vi "IHM_detection_powerSpectrum.vi"() -> ()   [LabVIEW 2009]
uses:
  <vilib>/Analysis/4window.llb/windowTd.ctl
  <vilib>/measure/maspectr.llb/FFT Power Spectrum for 1 Chan.vi
  <vilib>/measure/NI_MAPro.lvlib
  <vilib>/Analysis/NI_AALPro.lvlib
  <vilib>/Analysis/NI_AALBase.lvlib
panel:
  out "ModeMagnetude":T1(graph) caption="modeMagnetude"
  in  "intervals":i32=100 caption="intervalles"
  in  "background":bool
  out "backgroundSpectrum":dbl[](array[numeric])
  in  "averaging parameters":T2={"averaging mode"=enum."RMS averaging", "weighting mode"=enum."Linear", "number of averages"=10}
  in  "Freq.Bandwidth [%]":dbl
  in  "stop":bool
  out "averages completed":dbl caption="moyennes effectuées"
  out "averaging done":bool caption="moyennage terminé"
  out "RelativeMagnitude@Freq":dbl(graph)
  out "error out":errorcluster caption="sortie d'erreur"
  out "spectre":cluster{dbl[], "Data out":dbl[]}(graph)
  out "input signal":cluster{dbl[], "Data out":dbl[]}(graph)
  in  "attente (ms)":u32=10
  out "Freq. detected":bool
  in  "Frequency to detect [hz]":dbl=5000.0
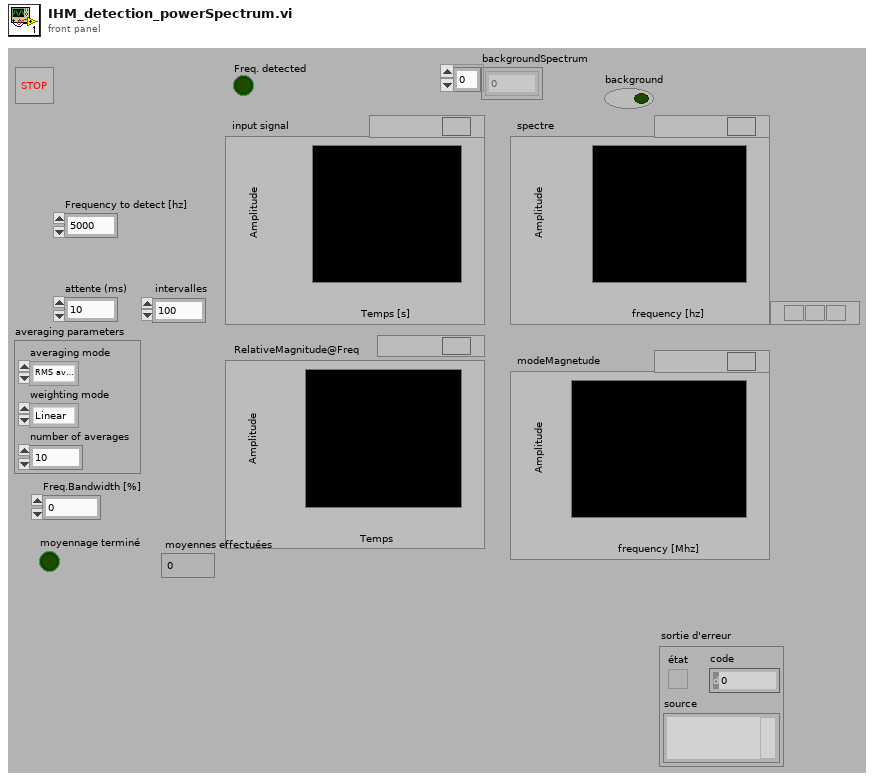
[diagram p1: front panel]
types:
  T1 = cluster{"X Values":dbl[], "Histogram: h(x)":i32[]}
  T2 = cluster{"averaging mode":enum16{"No averaging", "Vector averaging", "RMS averaging", "Peak hold"}, "weighting mode":enum16{"Linear", "Exponential"}, "number of averages":u32}
  T3 = typedef "NI_AALPro.lvlib/windowTd.ctl" = u32
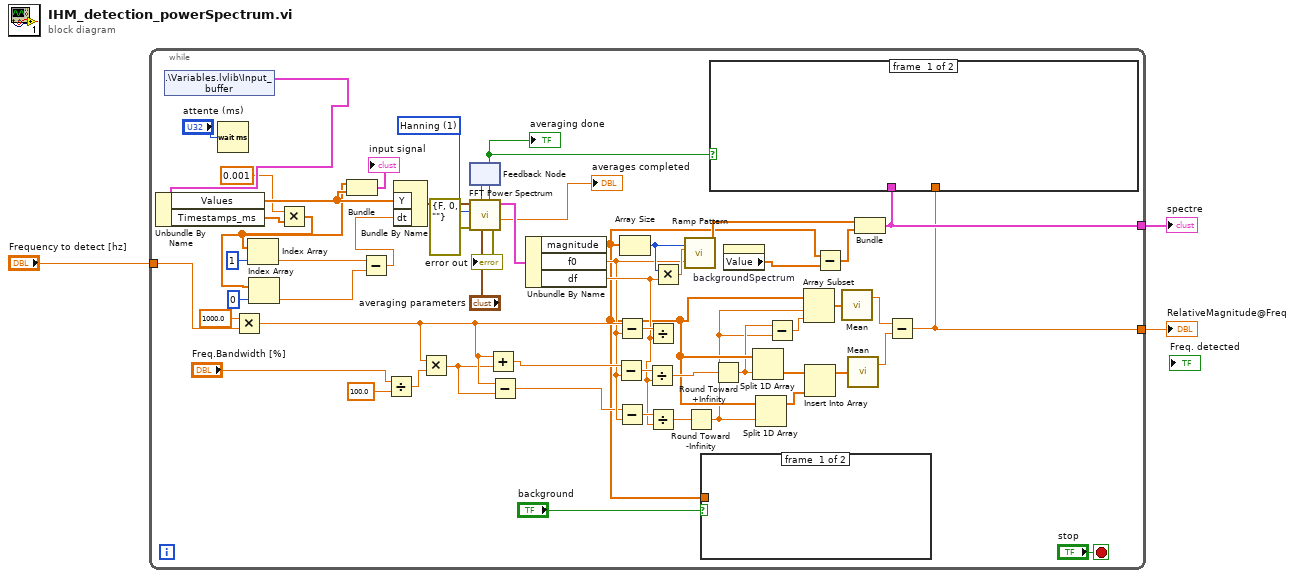
[diagram p0: block diagram]
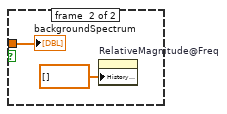
[diagram p2: hidden frame]
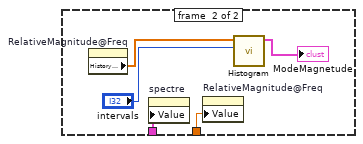
[diagram p3: hidden frame]
diagram:
  n1 = while {
    tunnel: "Frequency to detect [hz]" -> [w58]
    tunnel: [w45] -> w2
    tunnel: [w39] -> w1
    stop <- "stop" stop-if-true
    w53 = T3 1 items=["Rectangle"=0, "Hanning"=1, "Hamming"=2, "Blackman Harris"=3, "Blackman exacte"=4, "Blackman"=5, "Profil plat"=6, "B-Harris 4 termes "=7, "B-Harris 7 termes"=8, "Lobe latéral bas"=9, "Blackman Nuttall"=11, "Triangle"=30, "Bartlett-Hanning"=31, "Bohman"=32, "Parzen"=33, "Welch"=34, "Kaiser"=60, "Dolph-Tchebychev"=61, "Gaussienne"=62] ("window")
    n2 = shared-variable ".\\Variables.lvlib\\Input_buffer"() -> (w11:cluster{"Values":dbl[], "Timestamps_ms":dbl[]})  [unwired: 1 in, 1 out]
    n3 = Unbundle By Name(w11) -> ("Values"=w10:dbl[], "Timestamps_ms"=w5:dbl[])
    n4 = Wait (ms)(milliseconds to wait="attente (ms)") -> ()  [unwired: 1 out]
    n5 = Multiply(x=1000.0 ("y"), y=w58) -> (x*y=w32:dbl)
    n6 = Multiply(x=0.001, y=w5) -> (x*y=w4:dbl[])
    n7 = Index Array(array=w4, index=1 ("indice")) -> (element=w8:dbl)
    n8 = Index Array(array=w4, index=0 ("indice")) -> (element=w55:dbl)
    n9 = Bundle(w4, "Values"=w10) -> (→"input signal":cluster{dbl[], "Values":dbl[]})  [unwired: 1 in]
    n10 = Subtract(x=w8, y=w55) -> (x-y=w6:dbl)
    n11 = Divide(x="Freq.Bandwidth [%]", y=100.0) -> (x/y=w21:dbl)
    n12 = Bundle By Name("Y"=w10, "dt"=w6) -> (w54:waveform(dbl))  [unwired: 1 in]
    n13 = Multiply(x=w32, y=w21) -> (x*y=w31:dbl)
    n14 = feedback #1() -> (w44:bool)  [unwired: 1 in]
    n15 = call-poly <vilib>:"FFT Power Spectrum.vi"("averaging parameters"="averaging parameters", "restart averaging (F)"=w44, "error in (no error)"=errorcluster {"status"=FALSE, "code"=0, "source"=""}, "window"=w53, "time signal"=w54) -> ("error out"=→"error out":errorcluster, "averages completed"=→"averages completed":dbl, "power spectrum"=w52:cluster{"f0":dbl, "df":dbl, "magnitude":dbl[]}, "averaging done"=w43:bool)  [unwired: 3 in]
    "averaging done" <- w43
    n16 = Add(x=w32, y=w31) -> (x+y=w33:dbl)
    n17 = Subtract(x=w32, y=w31) -> (x-y=w27:dbl)
    n18 = Unbundle By Name(w52) -> ("magnitude"=w17:dbl[], "f0"=w28:dbl, "df"=w29:dbl)
    n19 = Subtract(x=w33, y=w28) -> (x-y=w40:dbl)
    n20 = Subtract(x=w32, y=w28) -> (x-y=w47:dbl)
    n21 = Subtract(x=w27, y=w28) -> (x-y=w30:dbl)
    n22 = Array Size(array=w17) -> (size(s)=w49:i32)
    n23 = Divide(x=w40, y=w29) -> (x/y=w19:dbl)
    n24 = Divide(x=w47, y=w29) -> ()  [unwired: 1 out]
    n25 = Divide(x=w30, y=w29) -> (x/y=w18:dbl)
    n26 = Multiply(x=w49, y=w29) -> (x*y=w48:dbl)
    n27 = call <vilib>:"Ramp Pattern.vi"("start"=w28, "end"=w48, "samples"=w49) -> ("Ramp Pattern"=w36:dbl[])  [unwired: 7 in, 1 out]
    n28 = Round Toward -Infinity(1:w18) -> (0:w13:dbl)
    n29 = case shown="Vrai" "background" {
      tunnel: w17 -> [_ w61]
      frame #0 {
      }
      frame #1 {
        n30 = property on="RelativeMagnitude@Freq" class="GraphDér (strict)"("History Data"=dbl[] [] ("Données d'historique")) -> ()  [unwired: 2 in, 2 out]
        "backgroundSpectrum" <- w61
      }
    }
    n31 = Round Toward +Infinity(x=w19) -> (ceil(x): smallest int >= x=w14:dbl)
    n32 = property on="backgroundSpectrum" class="Tabl (strict)"() -> ("Value"=w34:dbl[])  [unwired: 2 in, 2 out]
    n33 = Split 1D Array(array=w17, index=w14) -> (second subarray=w26:dbl[])  [unwired: 1 out]
    n34 = Split 1D Array(array=w17, index=w13) -> (first subarray=w25:dbl[])  [unwired: 1 out]
    n35 = Subtract(x=w14, y=w13) -> (x-y=w12:dbl)
    n36 = Array Subset(array=w17, index=w13, length=w12) -> (w16:dbl[])
    n37 = Insert Into Array(array=w26, new element=w25) -> (w24:dbl[])  [unwired: 1 in]
    n38 = Subtract(x=w17, y=w34) -> (x-y=w35:dbl[])
    n39 = call <vilib>:"Mean.vi"("X"=w16) -> ("mean"=w15:dbl)  [unwired: 1 out]
    n40 = call <vilib>:"Mean.vi"("X"=w24) -> ("mean"=w23:dbl)  [unwired: 1 out]
    n41 = Bundle("Ramp Pattern"=w36, w35) -> (w45:cluster{"Ramp Pattern":dbl[], dbl[]})  [unwired: 1 in]
    n42 = Subtract(x=w15, y=w23) -> (x-y=w39:dbl)
    n43 = case shown="Vrai" w43 {
      tunnel: w45 -> [_ w66]
      tunnel: w39 -> [_ w65]
      frame #0 {
      }
      frame #1 {
        n44 = property on="RelativeMagnitude@Freq" class="GraphDér (strict)"() -> ("History Data"=w64:dbl[])  [unwired: 2 in, 2 out]
        n45 = property on="spectre" class="GraphXY (strict)"("Value"=w66) -> ()  [unwired: 2 in, 2 out]
        n46 = property on="RelativeMagnitude@Freq" class="GraphDér (strict)"("Value"=w65) -> ()  [unwired: 2 in, 2 out]
        n47 = call <vilib>:"Histogram.vi"("intervals"="intervals", "X"=w64) -> ("Histogram Graph"=→"ModeMagnetude":T1)  [unwired: 6 in, 3 out]
      }
    }
  }
  "spectre" <- w2
  "RelativeMagnitude@Freq" <- w1
